vi "No Error.vi"() -> ()   [LabVIEW 2017, in "Transparent Assertions.Tests.lvlib" / "Assert Not Error.lvlib"]
uses:
  Assert Not Error.lvlib
  src/Transparent Assertions/Transparent Assertions.lvlib
panel:
  out "error out":errorcluster
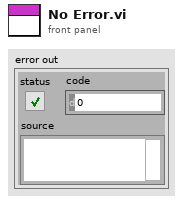
[diagram p1: front panel]
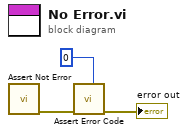
[diagram p0: block diagram]
diagram:
  n1 = call "Assert Not Error.vi"() -> ("error out"=w1:errorcluster)  [unwired: 11 in]
  n2 = call "Assert Error Code.vi"("Expected"=0, "error in (no error)"=w1) -> ("error out"=→"error out":errorcluster)  [unwired: 9 in]
